vi "fromCluster.vi"(8 "error in (no error)":errorcluster, 10 "ACNET Device Cluster":T1, 11 "ACNET Device in":refnum<class "ACNET Device.lvclass">) -> (0 "error out":errorcluster, 3 "ACNET Device out":refnum<class "ACNET Device.lvclass">)   [LabVIEW 2013, in "ACNET Monitor.lvlib" / "ACNET Device.lvclass"]
uses:
  ACNET Device.lvclass
  ACNET Device.lvclass/ACNET Device.ctl
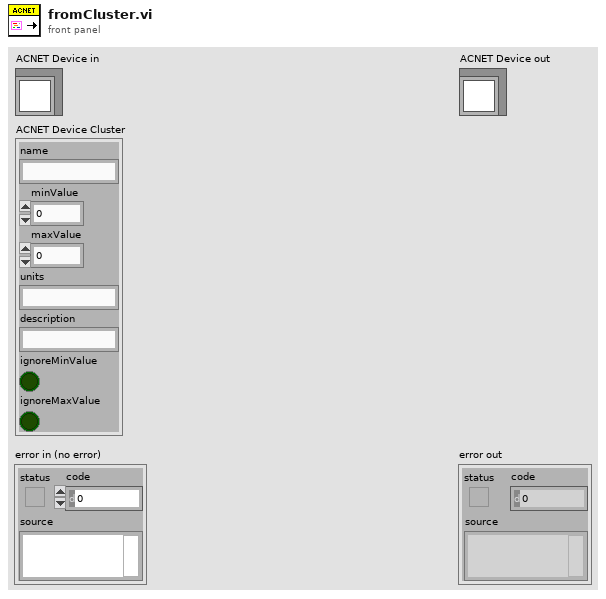
[diagram p1: front panel]
types:
  T1 = cluster{"name":string, "minValue":dbl, "maxValue":dbl, "units":string, "description":string, "ignoreMinValue":bool, "ignoreMaxValue":bool}
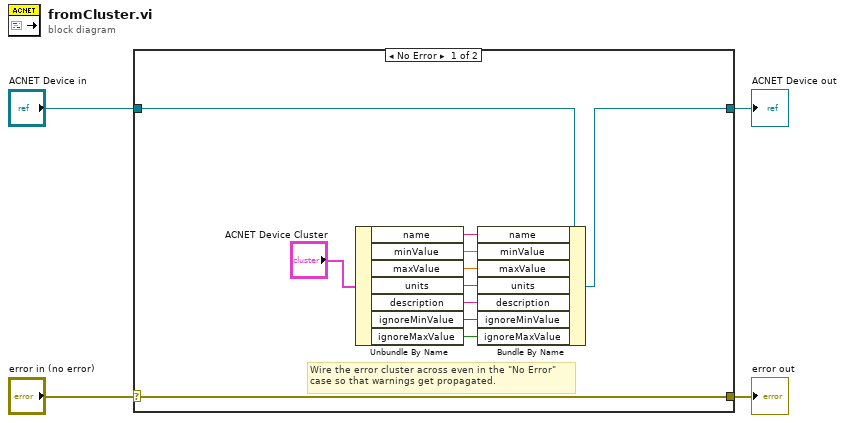
[diagram p0: block diagram]
diagram:
  n1 = case shown="No Error" "error in (no error)" {
    selector: "error in (no error)" -> [w8 w17]
    tunnel: [w8 w17] -> w3
    tunnel: [w9 w16] -> w1
    tunnel: "ACNET Device in" -> [w10 w16]
    frame No Error {
      # "Wire the error cluster across even in the \"No Error\"\ncase so that warnings get propagated."
      n2 = Unbundle By Name("ACNET Device Cluster") -> ("name"=w15:string, "minValue"=w14:dbl, "maxValue"=w13:dbl, "units"=w12:string, "description"=w7:string, "ignoreMinValue"=w6:bool, "ignoreMaxValue"=w5:bool)
      n3 = Bundle By Name(cluster=w10, "name"=w15, "minValue"=w14, "maxValue"=w13, "units"=w12, "description"=w7, "ignoreMinValue"=w6, "ignoreMaxValue"=w5) -> (w9:refnum<class "ACNET Device.lvclass">)
    }
    frame Error {
    }
  }
  "error out" <- w3
  "ACNET Device out" <- w1
